vi "aal_Complex Modulator(real input).vi"(1 "reset ?":bool, 2 "fs":dbl=1024.0 min=-0.5 max=0.5 format="%.2f", 3 "frequency":dbl min=-0.5 max=0.5 format="%.2f", 4 "x":dbl[](array[numeric])) -> (0 "y":cdb[](array[numeric]))   [LabVIEW 2014, in "NI_AALPro.lvlib"]
doc: "Modulates the signal to frequency. The center frequency should be normalized (-0.5, 0.5)."
uses:
  NI_AALPro.lvlib
  lvanlys.dll
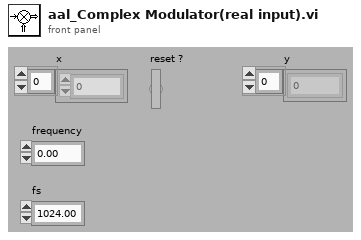
[diagram p1: front panel]
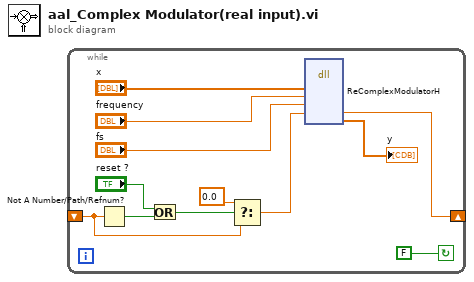
[diagram p0: block diagram]
diagram:
  n1 = while {
    shift-left: _ -> [w10]
    shift-right: [w5] -> _
    stop <- FALSE continue-if-true
    n2 = Not A Number/Path/Refnum?(number/path/refnum=w10) -> (NaN/Path/Refnum?=w12:bool)
    n3 = Or(x="reset ?", y=w12) -> (x .or. y?=w4:bool)
    n4 = Select(t=0.0, s=w4, f=w10) -> (s? t:f=w6:dbl)
    n5 = dll-call lib="C:/Program Files (x86)/National Instruments/LabVIEW 2014/resource/lvanlys.*" fn="ReComplexModulatorH"("x"="x", "fc"="frequency", "fs"="fs", "initial_phase"=w6) -> ("initial_phase"=w5:dbl, "y"=→"y":cdb[])  [unwired: 8 in, 2 out]
  }
